vi "loop-while-switch-case.vi"() -> ()   [LabVIEW 2026]
panel:
  in  "Boolean":bool
  out "Contador":i32
  out "°C":dbl(slide) scale=0.0..100.0
  out "Conversão part. 1":dbl
  in  "°F":dbl(slide) scale=0.0..273.0
  in  "stop":bool
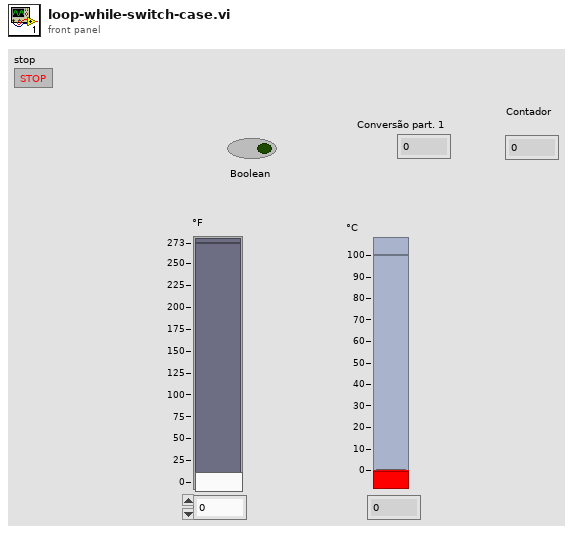
[diagram p1: front panel]
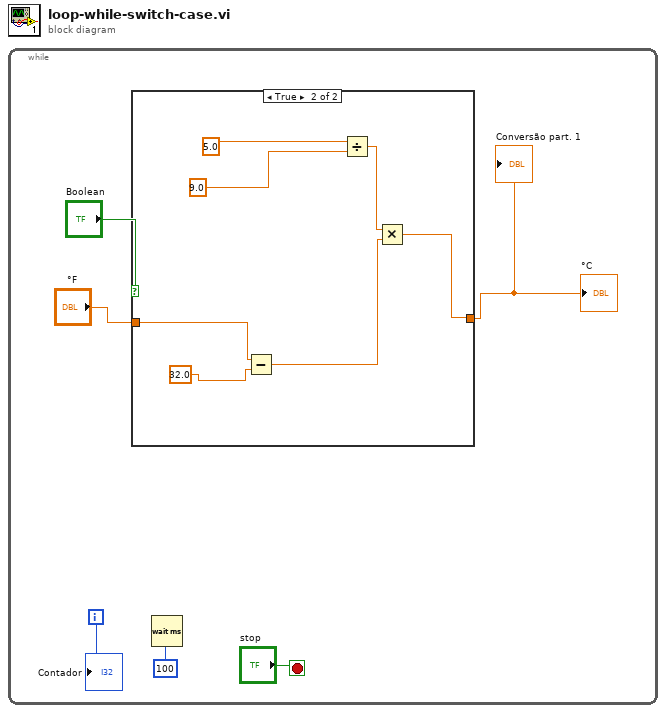
[diagram p0: block diagram]
diagram:
  n1 = while {
    i -> [w4]
    stop <- "stop" stop-if-true
    n2 = case shown="True" "Boolean" {
      tunnel: "°F" -> [w7 w11]
      tunnel: [w7 w8] -> w5
      frame False {
      }
      frame True {
        n3 = Subtract(x=w11, y=32.0) -> (x-y=w9:dbl)
        n4 = Divide(x=5.0, y=9.0) -> (x/y=w12:dbl)
        n5 = Multiply(x=w12, y=w9) -> (x*y=w8:dbl)
      }
    }
    "Conversão part. 1" <- w5
    "°C" <- w5
    n6 = Wait (ms)(milliseconds to wait=u32 100) -> ()  [unwired: 1 out]
    "Contador" <- w4
  }
